vi "LED-Global-string-length.vi"() -> ()   [LabVIEW 2020]
panel:
  out "LED STRING LENGTH":dbl=60.0
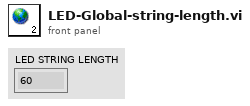
[diagram p1: front panel]
diagram:
